vi "Load Conditions.vi"(6 "Constants":refnum<class "Sequence Constants.lvclass">, 8 "error in (no error)":refnum<class "MultiErrors.lvclass">, 10 "Config Element":refnum<class "Config Element.lvclass">) -> (0 "error out":refnum<class "MultiErrors.lvclass">, 2 "Conditions":refnum<class "Condition Config.lvclass">[](array[class]))   [LabVIEW 2020, in "VolatusSeqConfig.lvlib" / "Transition Config.lvclass"]
uses:
  Transition Config.lvclass
  lv-cdm/CDM-Config/Config Element/Config Element.lvclass
  Condition Config/Condition Config.lvclass
  VolatusErrorUtilities/MultiErrors/MultiErrors.lvclass
  VolatusErrorUtilities/MultiErrors/MultiErrors.lvclass/MultiErrors.ctl
  Transition Config.lvclass/Transition Config.ctl
  VolatusSeqConfig.lvlib
  Sequence Constants/Sequence Constants.lvclass
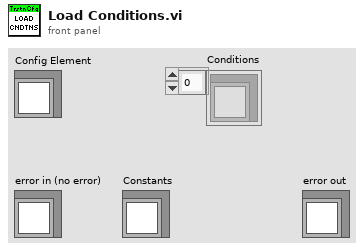
[diagram p1: front panel]
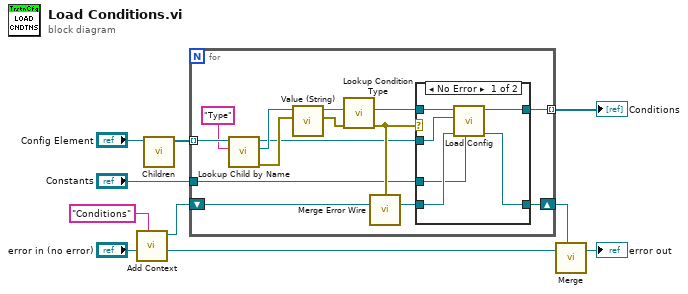
[diagram p0: block diagram]
diagram:
  n1 = call "Add Context.vi"("Context"="Conditions", "MultiErrors in"="error in (no error)") -> ("Original Context"=w4:refnum<class "MultiErrors.lvclass">, "Added Context"=w5:refnum<class "MultiErrors.lvclass">)  [unwired: 8 in]
  n2 = call "Children.vi"("Config Element in"="Config Element") -> ("Elements"=w9:refnum<class "Config Element.lvclass">[])  [unwired: 9 in, 1 out]
  n3 = for {
    tunnel: w9 -> [w22] mode=indexing
    tunnel: [w15] -> w8 mode=indexing
    shift-right: [w12] -> w2
    shift-left: w5 -> [w14]
    tunnel: "Constants" -> [w11]
    n4 = call "Lookup Child by Name.vi"("Name"="Type", "Config Element in"=w22) -> ("error out"=w24:errorcluster, "Child"=w20:refnum<class "Config Element.lvclass">, "Config Element out"=w16:refnum<class "Config Element.lvclass">)  [unwired: 6 in, 1 out]
    n5 = call "Value (String).vi"("error in (no error)"=w24, "Config Element in"=w20) -> ("error out"=w18:errorcluster, "String Value"=w19:string)  [unwired: 8 in]
    n6 = call "Lookup Condition Type.vi"("error in (no error)"=w18, "Condition Type"=w19) -> ("error out"=w23:errorcluster, "Condition"=w17:refnum<class "Condition Config.lvclass">)  [unwired: 8 in]
    n7 = call "Merge Error Wire.vi"("error in (no error)"=w23, "MultiErrors in"=w14) -> ("MultiErrors out"=w13:refnum<class "MultiErrors.lvclass">)  [unwired: 13 in]
    n8 = case shown="No Error" w23 {
      tunnel: w17 -> [w30 _]
      tunnel: w16 -> [w29 _]
      tunnel: [w28 _] -> w15
      tunnel: w13 -> [w27 w31]
      tunnel: [w26 w31] -> w12
      tunnel: w11 -> [w25 _]
      frame No Error {
        n9 = call-dynamic "Load Config.vi"("Constants"=w25, "error in (no error)"=w27, "Config Element"=w29, "Condition Config in"=w30) -> ("error out"=w26:refnum<class "MultiErrors.lvclass">, "Condition Config out"=w28:refnum<class "Condition Config.lvclass">)  [unwired: 6 in]
      }
      frame Error {
      }
    }
  }
  "Conditions" <- w8
  n10 = call "Merge.vi"("First Error In"=w4, "Second Error In"=w2) -> ("MultiErrors out"=→"error out":refnum<class "MultiErrors.lvclass">)  [unwired: 5 in]
